vi "follow autonomous.vi"(0 "x":dbl, 1 "y":dbl, 4 "robot x":dbl, 5 "robot y":dbl, 6 "robot angle":dbl, 7 "speed kp":dbl, 9 "v":dbl) -> (19 "newV":dbl)   [LabVIEW 2016]
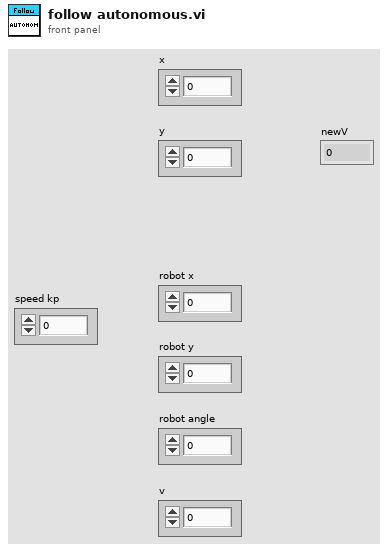
[diagram p1: front panel]
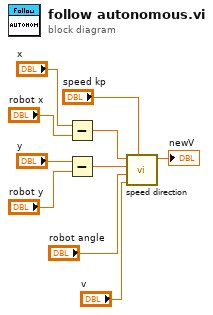
[diagram p0: block diagram]
diagram:
  n1 = Subtract(x="x", y="robot x") -> (x-y=w10:dbl)
  n2 = Subtract(x="y", y="robot y") -> (x-y=w9:dbl)
  n3 = call "speed direction.vi"("kp"="speed kp", "v"="v", "theta"="robot angle", "delta y"=w9, "delta x"=w10) -> ("newV"=→"newV":dbl)  [unwired: 6 in]
